vi "data_processing.vi"(11 "data":dynamicdata(waveform)) -> (3 "DATA":dbl[](array[numeric]))   [LabVIEW 2017]
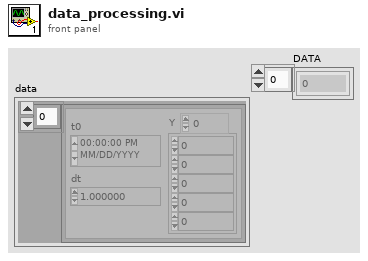
[diagram p1: front panel]
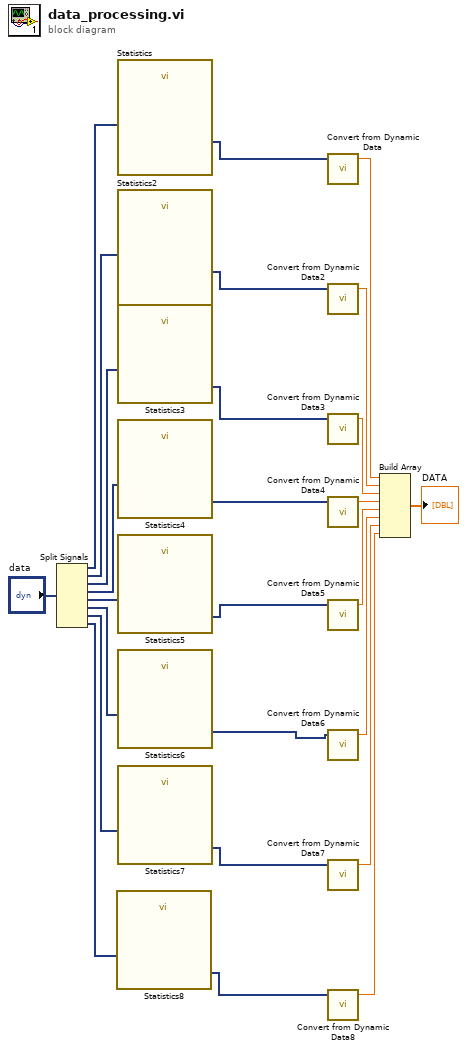
[diagram p0: block diagram]
diagram:
  n1 = Split Signals("data") -> (w25:dynamicdata, w24:dynamicdata, w23:dynamicdata, w22:dynamicdata, w21:dynamicdata, w20:dynamicdata, w19:dynamicdata, w18:dynamicdata)  [unwired: 8 in]
  n2 = call "Statistics8"("Signals"=w18) -> ("Arithmetic Mean"=w1:dynamicdata)  [unwired: 25 in, 1 out]
  n3 = call "Statistics"("Signals"=w25) -> ("Arithmetic Mean"=w8:dynamicdata)  [unwired: 25 in, 1 out]
  n4 = call "Statistics2"("Signals"=w24) -> ("Arithmetic Mean"=w7:dynamicdata)  [unwired: 25 in, 1 out]
  n5 = call "Statistics3"("Signals"=w23) -> ("Arithmetic Mean"=w6:dynamicdata)  [unwired: 25 in, 1 out]
  n6 = call "Statistics4"("Signals"=w22) -> ("Arithmetic Mean"=w5:dynamicdata)  [unwired: 25 in, 1 out]
  n7 = call "Statistics5"("Signals"=w21) -> ("Arithmetic Mean"=w4:dynamicdata)  [unwired: 25 in, 1 out]
  n8 = call "Statistics6"("Signals"=w20) -> ("Arithmetic Mean"=w3:dynamicdata)  [unwired: 25 in, 1 out]
  n9 = call "Statistics7"("Signals"=w19) -> ("Arithmetic Mean"=w2:dynamicdata)  [unwired: 25 in, 1 out]
  n10 = call "Convert from Dynamic Data"("Dynamic Data Type"=w8) -> ("Scalar"=w17:dbl)  [unwired: 3 in]
  n11 = call "Convert from Dynamic Data2"("Dynamic Data Type"=w7) -> ("Scalar"=w16:dbl)  [unwired: 3 in]
  n12 = call "Convert from Dynamic Data3"("Dynamic Data Type"=w6) -> ("Scalar"=w15:dbl)  [unwired: 3 in]
  n13 = call "Convert from Dynamic Data4"("Dynamic Data Type"=w5) -> ("Scalar"=w14:dbl)  [unwired: 3 in]
  n14 = call "Convert from Dynamic Data5"("Dynamic Data Type"=w4) -> ("Scalar"=w13:dbl)  [unwired: 3 in]
  n15 = call "Convert from Dynamic Data6"("Dynamic Data Type"=w3) -> ("Scalar"=w12:dbl)  [unwired: 3 in]
  n16 = call "Convert from Dynamic Data7"("Dynamic Data Type"=w2) -> ("Scalar"=w11:dbl)  [unwired: 3 in]
  n17 = call "Convert from Dynamic Data8"("Dynamic Data Type"=w1) -> ("Scalar"=w10:dbl)  [unwired: 3 in]
  n18 = Build Array(w17, w16, w15, w14, w13, w12, w11, w10) -> (→"DATA":dbl[])
